vi "LIA Example Host_v1.vi"() -> ()   [LabVIEW 2017]
uses:
  Program Files (x86)/National Instruments/LabVIEW 2017/examples/Lock-In Amplifier/lib/host/Public/pll settings.ctl
  Program Files (x86)/National Instruments/LabVIEW 2017/examples/Lock-In Amplifier/lib/host/Public/lock-in settings.ctl
  Program Files (x86)/National Instruments/LabVIEW 2017/examples/Lock-In Amplifier/lib/interface/Interface FPGA/LIA Host Interface FPGA.lvclass
  C:/Program Files (x86)/National Instruments/LabVIEW 2017/examples/Lock-In Amplifier/lib/interface/Interface/LIA Host Interface.lvclass
  Program Files (x86)/National Instruments/LabVIEW 2017/examples/Lock-In Amplifier/lib/host/Public/fpga type.ctl
  Program Files (x86)/National Instruments/LabVIEW 2017/examples/Lock-In Amplifier/lib/interface/Interface FPGA/Properties/FpgaSession_GET.vi
  <vilib>/Utility/error.llb/Error Cluster From Error Code.vi
  <vilib>/rvi/errors/niLvFpgaAdjustHostInterfaceError.vi
  <vilib>/rvi/interface/nirviReadWriteControl/nirviReadWriteControl.xnode
  Program Files (x86)/National Instruments/LabVIEW 2017/examples/Lock-In Amplifier/lib/interface/Interface/LIA Host Interface.lvclass
  Program Files (x86)/National Instruments/LabVIEW 2017/examples/Lock-In Amplifier/lib/host/Lock-In Amplifier Example Host.lvlib
  Program Files (x86)/National Instruments/LabVIEW 2017/examples/Lock-In Amplifier/lib/shared/Lock-In Amplifier Example Shared.lvlib
  NiFpgaLv.dll
  <vilib>/rvi/interface/Simulation/niFpgaSimulationCallBeginRW.vi
panel:
  out "lock-in.max-min":dbl=7.228629495115158e-05 caption="Deviation" format="%#_6p"
  out "lock-in.max 0":dbl=0.9100438567932344 caption="Deviation" format="%#_6p"
  out "lock-in.min 0":dbl=0.9099715704982833 caption="Deviation" format="%#_6p"
  out "# of IQ samples":i32=4096 caption="Result"
  out "Waveform Chart":cluster{"mean":dbl, "trace":dbl}(graph)={"mean"=0.9100080307156506, "trace"=0.9100209129308812}
  out "Waveform Graph":cluster{"f0":dbl, "df":dbl, "magnitude":dbl[]}[](graph)
  in  "trigger slope 1":enum16{"Positive", "Negative"}(ring)
  in  "lowLevel 1":dbl caption="pll.q 2" format="%#_6f"
  in  "highLevel 1":dbl=0.25 caption="pll.q 2" format="%#_6f"
  in  "trigger slope 0":enum16{"Positive", "Negative"}(ring)
  in  "lowLevel 0":dbl caption="pll.q 2" format="%#_6f"
  in  "highLevel 0":dbl=0.25 caption="pll.q 2" format="%#_6f"
  out "pll.vco output 0":fxp<+/-,49,1>=0.001000059403974518 format="%0^#1_8g"
  out "pll.q 2":dbl=100005.9403974518 format="%#_6pV"
  in  "app.quit":bool
  in  "lock-in.boxcar length 0":u32=2048 caption="Boxar Length"
  in  "app.tab 0":enum32{"Lock-In", "PLL", "Output"}(tab)
  in  "lock-in.manual carrier 0":dbl=100000.0 caption="Carrier" format="%#_6p"
  in  "lock-in.decimation 0":i32=1000 caption="Decimation" min=8 max=16384
  in  "lock-in.source 0":enum16{"AI 0", "AI 1", "AI 2", "AI 3"}(ring)=enum."AI 1" caption="Channel"
  in  "lock-in.carrier 0":T1(ring)=enum."PLL 0" caption="Carrier Source"
  in  "pll.m 0":i8=-27 caption="M"
  in  "pll.source 0":enum16{"AI 0", "AI 1", "AI 2", "AI 3"}(ring) caption="Source"
  in  "pll.q frequency 0":dbl=100000.0 caption="Q Frequency" format="%#_6p"
  in  "pll.reset 0":bool
  in  "ao.noise 3":dbl caption="A0 3 Noise" min=0.0 max=1.0 format="%#_6p"
  in  "ao.level 3":dbl caption="A0 3 Level" format="%#_6pV"
  in  "ao.frequency 3":dbl=10000000.0 caption="AO 3 Frequency" format="%#.9p"
  in  "ao.frequency 0":dbl=10000000.0 caption="AO 0 Frequency" format="%#.9p"
  in  "ao.level 0":dbl caption="AO 0 Level" format="%#_6pV"
  in  "rio device":tag="PXI1Slot8" caption="Resource"
  in  "lock-in.reset boxar 0":bool
  out "lock-in.deviation 0":dbl=2.8087799509727284e-06 caption="Deviation" format="%#_6p"
  out "lock-in.amplitude 0":dbl=0.9100080307156506 caption="Result" format="%#_6p"
  in  "lock-in.boxcar lookback 0":i32=1024 caption="Windows to Average"
  # "pll.digital config 0"
  # "pll.digital config 1"
  # "NI Lock-In Amplifier Reference Example"
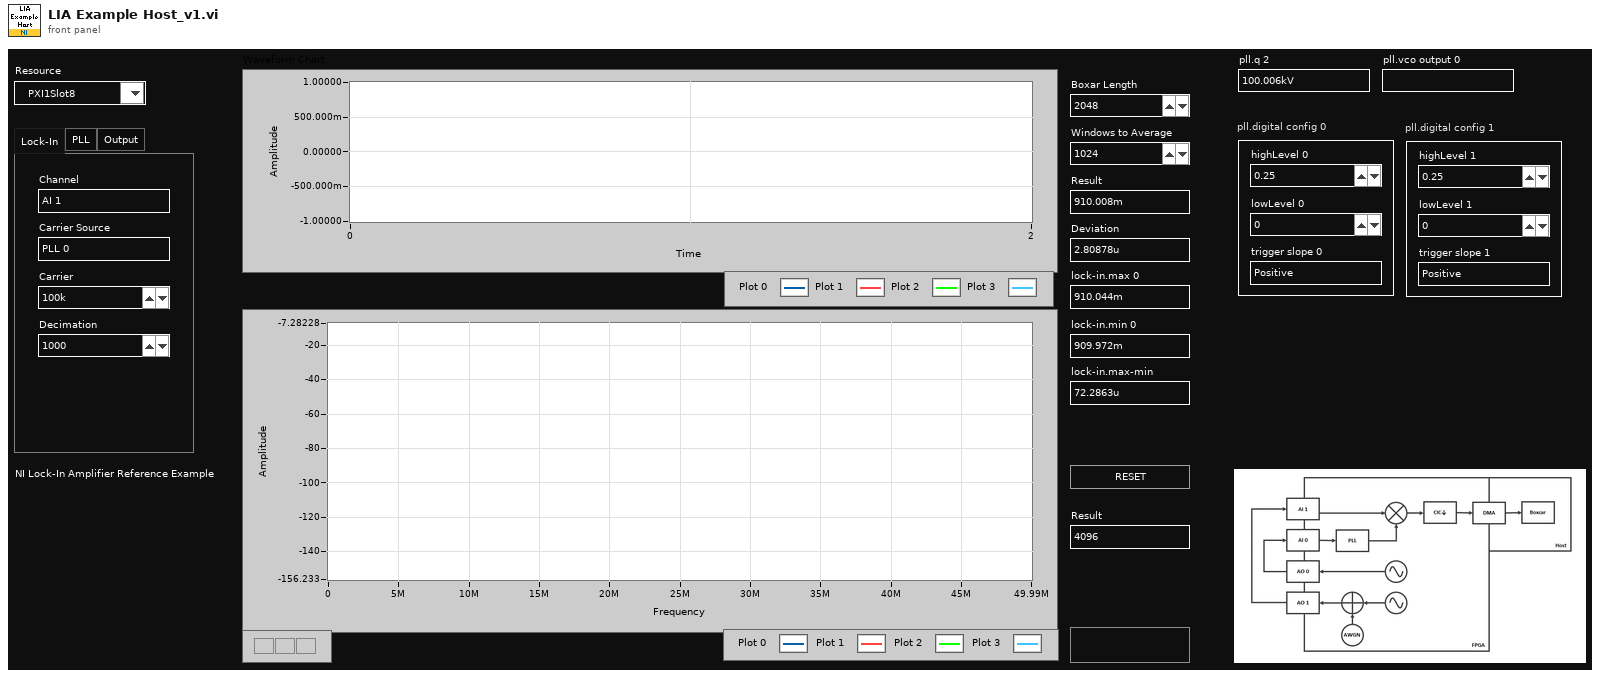
[diagram p1: front panel]
types:
  T1 = enum16{"Manual 0", "Manual 1", "Manual 2", "Manual 3", "PLL 0", "PLL 1"}
  T2 = typedef "Lock-In Amplifier Example Host.lvlib/lock-in settings.ctl" = cluster{"decimation":i32, "source":i32, "carrier source":i32, "carrier":dbl}
  T3 = typedef "Lock-In Amplifier Example Host.lvlib/pll settings.ctl" = cluster{"source":i32, "q frequency":dbl}
  T4 = cluster{"highLevel":fxp<+/-,18,1>, "lowLevel":fxp<+/-,18,1>, "trigger slope":enum8{"Positive", "Negative"}}
  T5 = typedef "Lock-In Amplifier Example Host.lvlib/fpga type.ctl" = refnum<k20>
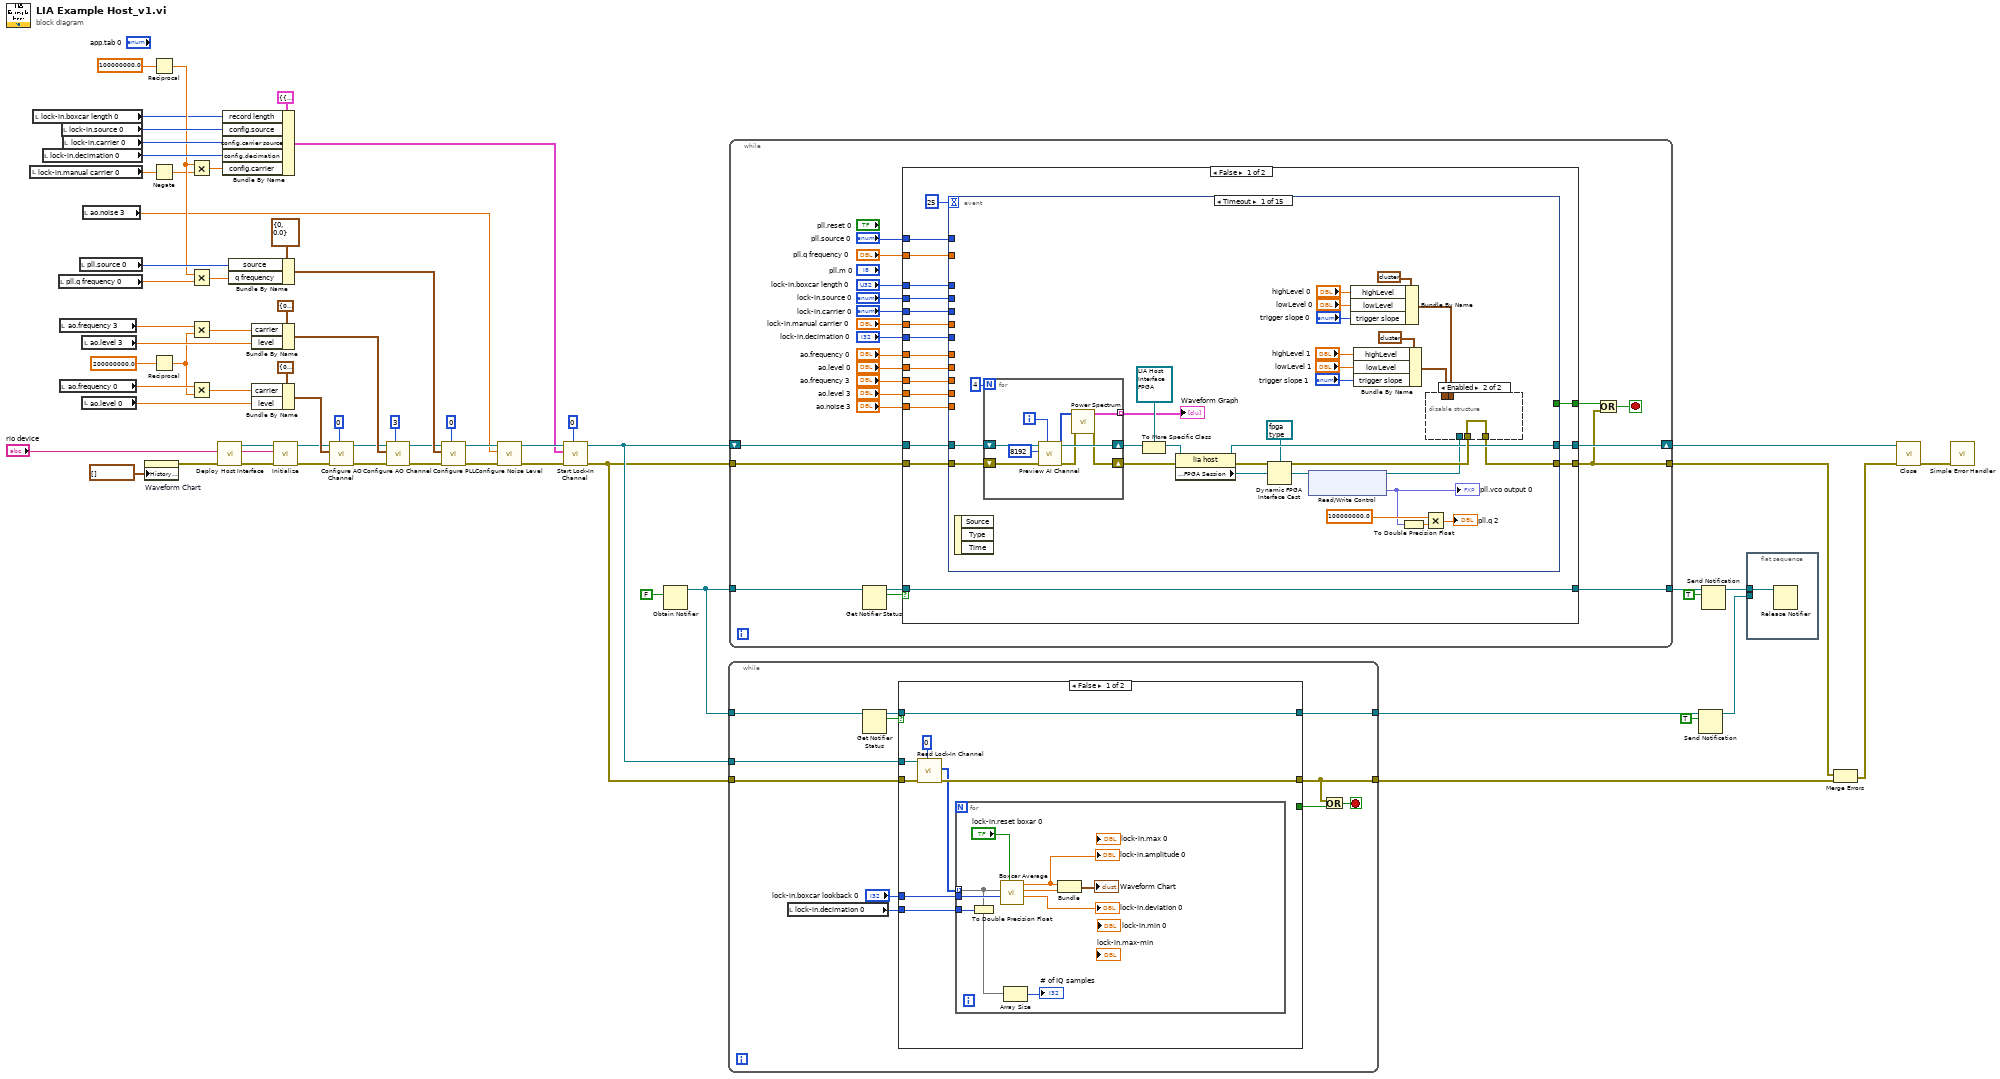
[diagram p0: block diagram]
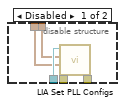
[diagram p2: hidden frame]
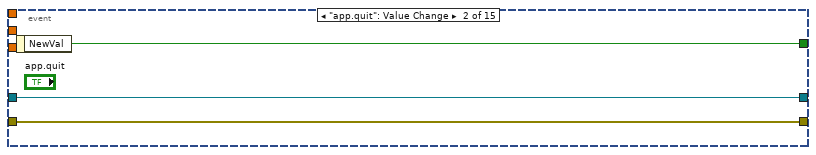
[diagram p3: hidden frame]
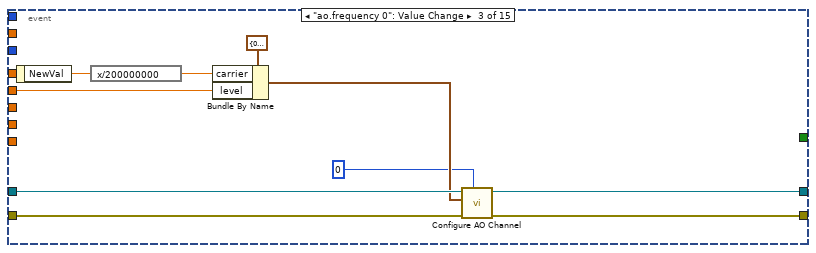
[diagram p4: hidden frame]
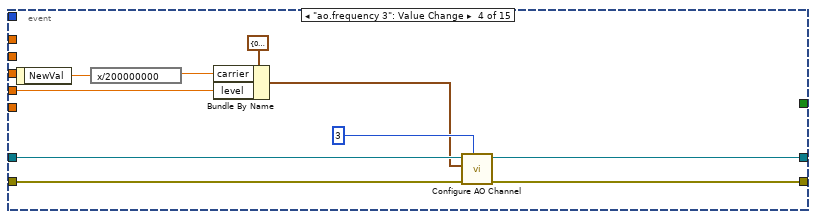
[diagram p5: hidden frame]
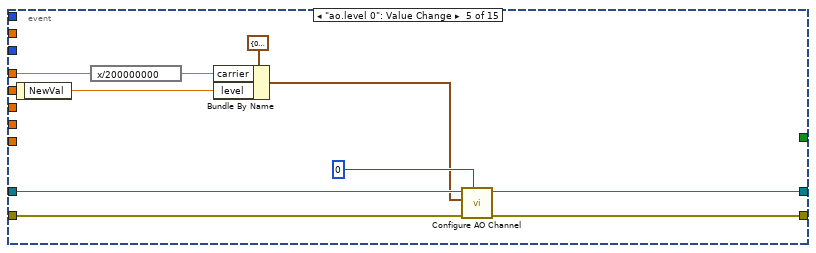
[diagram p6: hidden frame]
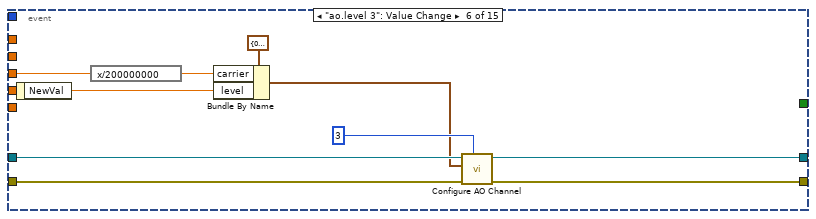
[diagram p7: hidden frame]
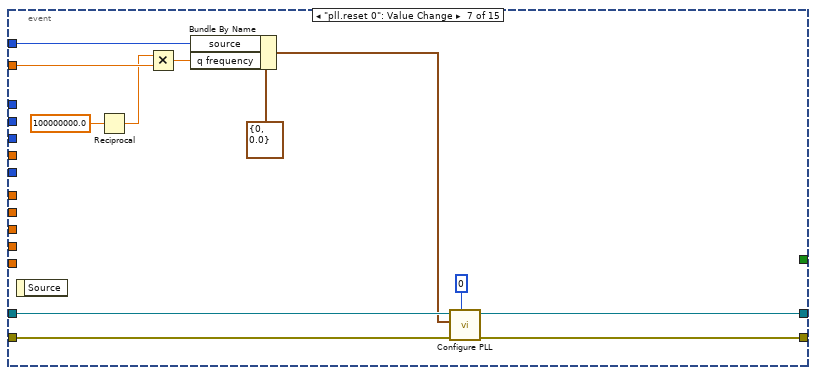
[diagram p8: hidden frame]
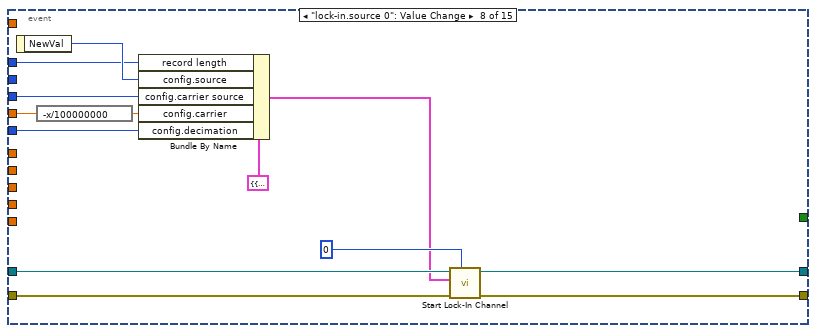
[diagram p9: hidden frame]
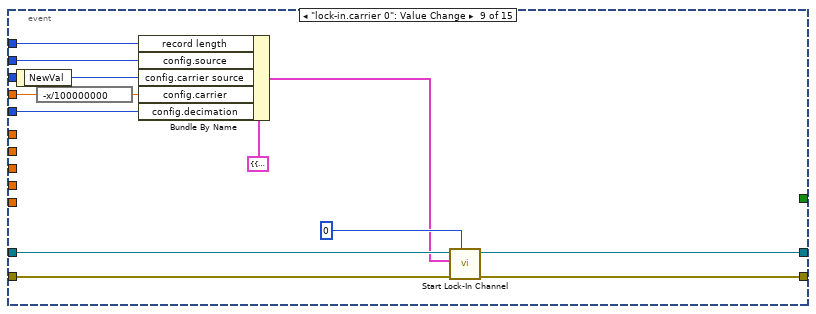
[diagram p10: hidden frame]
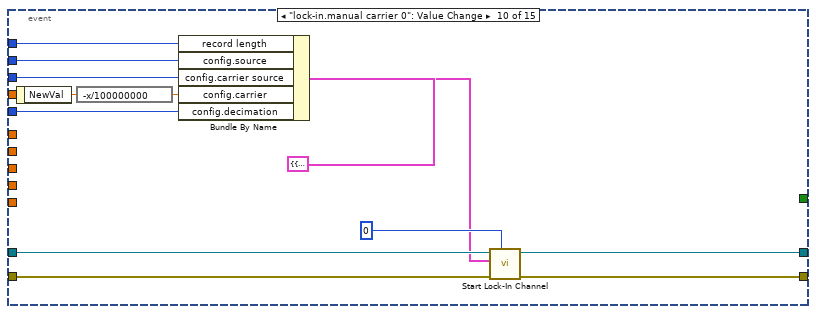
[diagram p11: hidden frame]
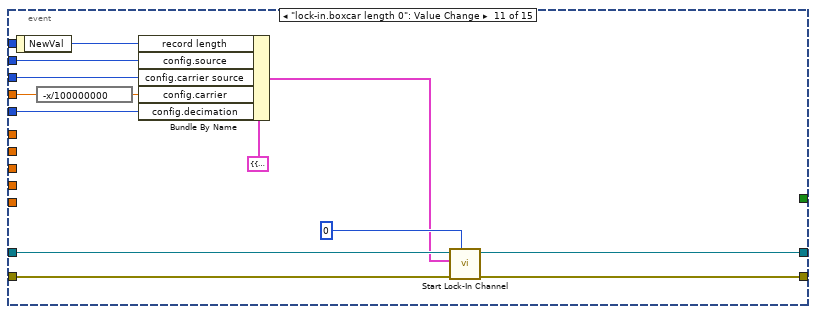
[diagram p12: hidden frame]
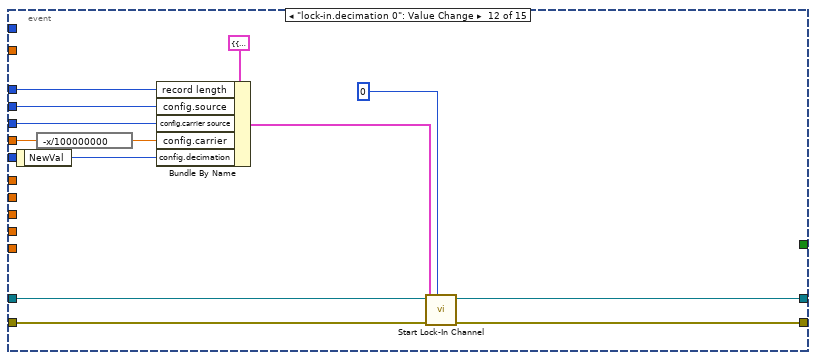
[diagram p13: hidden frame]
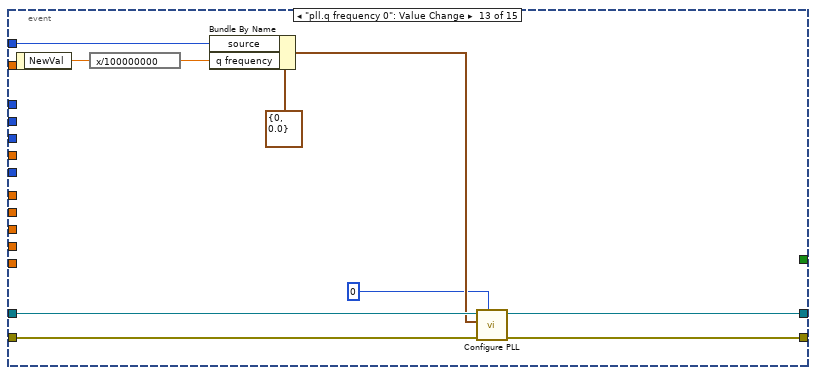
[diagram p14: hidden frame]
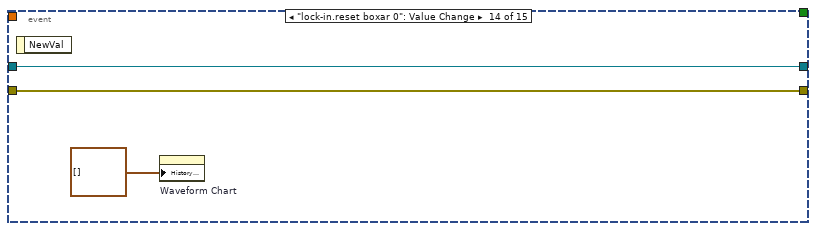
[diagram p15: hidden frame]
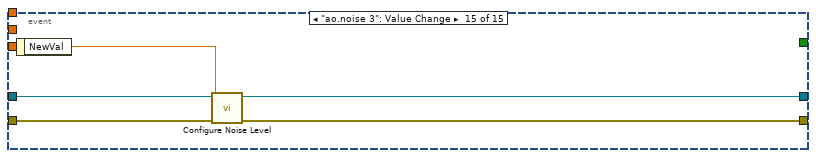
[diagram p16: hidden frame]
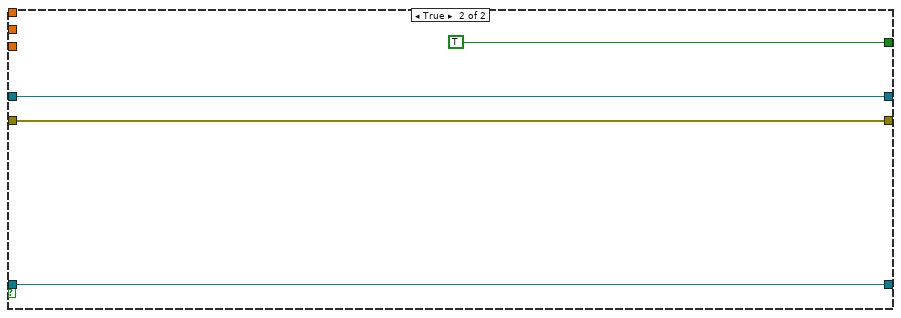
[diagram p17: hidden frame]
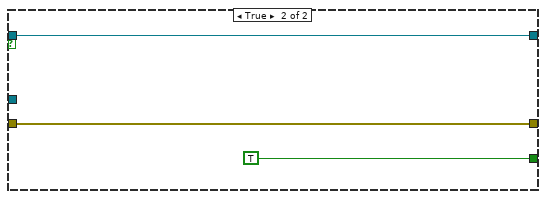
[diagram p18: hidden frame]
diagram:
  n1 = local read "lock-in.manual carrier 0"() -> (w50:dbl)
  n2 = local read "lock-in.boxcar length 0"() -> (w15:u32)
  n3 = local read "lock-in.decimation 0"() -> (w53:i32)
  n4 = local read "pll.q frequency 0"() -> (w55:dbl)
  n5 = local read "ao.frequency 3"() -> (w47:dbl)
  n6 = local read "ao.frequency 0"() -> (w44:dbl)
  n7 = local read "lock-in.source 0"() -> (w64:enum16{"AI 0", "AI 1", "AI 2", "AI 3"})
  n8 = local read "lock-in.carrier 0"() -> (w63:T1)
  n9 = local read "pll.source 0"() -> (w61:enum16{"AI 0", "AI 1", "AI 2", "AI 3"})
  n10 = local read "ao.level 3"() -> (w59:dbl)
  n11 = local read "ao.level 0"() -> (w58:dbl)
  n12 = local read "ao.noise 3"() -> (w6:dbl)
  n13 = property on="Waveform Chart" class="WFChart (strict)"("History Data"=cluster{"mean":dbl, "trace":dbl}[] []) -> (error out=w2:errorcluster)  [unwired: 2 in, 1 out]
  n14 = Reciprocal(x=100000000.0) -> (1/x=w51:dbl)
  n15 = Negate(x=w50) -> (-x=w49:dbl)
  n16 = Reciprocal(x=200000000.0) -> (1/x=w43:dbl)
  n17 = Multiply(x=w51, y=w49) -> (x*y=w52:dbl)
  n18 = Multiply(x=w51, y=w55) -> (x*y=w56:dbl)
  n19 = Multiply(x=w47, y=w43) -> (x*y=w48:dbl)
  n20 = Multiply(x=w44, y=w43) -> (x*y=w45:dbl)
  n21 = call "Deploy Host Interface.vi"("error in"=w2, "resource"="rio device") -> ("error out"=w11:errorcluster, "resource out"=w12:string, "lia host interface"=w13:refnum<class "LIA Host Interface.lvclass">)  [unwired: 7 in]
  n22 = Bundle By Name(cluster=cluster{"config":T2, "record length":u32} {"config"={"decimation"=0, "source"=0, "carrier source"=0, "carrier"=0.0}, "record length"=0} ("config"), "record length"=w15, "config.source"=w64, "config.carrier source"=w63, "config.decimation"=w53, "config.carrier"=w52) -> (w1:cluster{"config":T2, "record length":u32})
  n23 = Bundle By Name(cluster=T3 {"source"=0, "q frequency"=0.0} ("config"), "source"=w61, "q frequency"=w56) -> (w40:T3)
  n24 = Bundle By Name(cluster=cluster{"carrier":dbl, "level":dbl} {"carrier"=0.0, "level"=0.0} ("config"), "carrier"=w48, "level"=w59) -> (w41:cluster{"carrier":dbl, "level":dbl})
  n25 = Bundle By Name(cluster=cluster{"carrier":dbl, "level":dbl} {"carrier"=0.0, "level"=0.0} ("config"), "carrier"=w45, "level"=w58) -> (w42:cluster{"carrier":dbl, "level":dbl})
  n26 = call-dynamic "Initialize.vi"("error in"=w11, "resource"=w12, "lia host in"=w13) -> ("error out"=w24:errorcluster, "lia host out"=w25:refnum<class "LIA Host Interface.lvclass">)  [unwired: 7 in]
  n27 = call-dynamic "Configure AO Channel.vi"("instance"=0 ("index"), "error in"=w24, "config"=w42, "lia host in"=w25) -> ("error out"=w23:errorcluster, "lia host out"=w22:refnum<class "LIA Host Interface.lvclass">)  [unwired: 6 in]
  n28 = call-dynamic "Configure AO Channel.vi"("instance"=3 ("index"), "error in"=w23, "config"=w41, "lia host in"=w22) -> ("error out"=w18:errorcluster, "lia host out"=w19:refnum<class "LIA Host Interface.lvclass">)  [unwired: 6 in]
  n29 = call-dynamic "Configure PLL.vi"("instance"=0 ("index"), "error in"=w18, "config"=w40, "lia host in"=w19) -> ("error out"=w10:errorcluster, "lia host out"=w7:refnum<class "LIA Host Interface.lvclass">)  [unwired: 6 in]
  n30 = call-dynamic "Configure Noise Level.vi"("error in"=w10, "level"=w6, "lia host in"=w7) -> ("error out"=w9:errorcluster, "lia host out"=w8:refnum<class "LIA Host Interface.lvclass">)  [unwired: 7 in]
  n31 = call-dynamic "Start Lock-In Channel.vi"("instance"=0 ("index"), "error in"=w9, "config"=w1, "lia host in"=w8) -> ("error out"=w35:errorcluster, "lia host out"=w36:refnum<class "LIA Host Interface.lvclass">)  [unwired: 6 in]
  n32 = Obtain Notifier(notification data type=FALSE) -> (notifier out=w37:refnum<notifier>)  [unwired: 3 in, 2 out]
  n33 = while {
    tunnel: w37 -> [w75]
    tunnel: w36 -> [w72]
    tunnel: w35 -> [w71]
    tunnel: [w70] -> w28
    tunnel: [w67] -> w31
    stop <- w69 stop-if-true
    n34 = local read "lock-in.decimation 0"() -> (w65:i32)
    n35 = Get Notifier Status(notifier=w75) -> (notifier out=w73:refnum<notifier>, current notification=w74:bool)  [unwired: 1 in, 3 out]
    n36 = case shown="False" w74 {
      tunnel: [w80 w95] -> w67
      tunnel: w73 -> [w80 w95]
      tunnel: w72 -> [w83 _]
      tunnel: w71 -> [w82 w94]
      tunnel: [w79 w94] -> w70
      tunnel: [_ TRUE] -> w68
      tunnel: "lock-in.boxcar lookback 0" -> [w78 _]
      tunnel: w65 -> [w76 _]
      frame False {
        n37 = call-dynamic "Read Lock-In Channel.vi"("instance"=0 ("index"), "error in"=w82, "lia host in"=w83) -> ("error out"=w79:errorcluster, "unscaled data"=w77:i64[][])  [unwired: 6 in, 1 out]
        n38 = for {
          tunnel: w77 -> [w85] mode=indexing
          tunnel: w78 -> [w90]
          tunnel: w76 -> [w84]
          n39 = To Double Precision Float(number=w84) -> ()  [unwired: 1 out]
          n40 = call "Boxcar Average.vi"("reset"="lock-in.reset boxar 0", "sample length"=w90, "interleaved iq"=w85) -> ("standard deviation"=→"lock-in.deviation 0":dbl, "trace"=w87:dbl, "mean"=w91:dbl)  [unwired: 6 in]
          "lock-in.amplitude 0" <- w91
          n41 = Array Size(array=w85) -> (size(s)=→"# of IQ samples":i32)
          n42 = Bundle("mean"=w91, "trace"=w87) -> (→"Waveform Chart":cluster{"mean":dbl, "trace":dbl})  [unwired: 1 in]
        }
      }
      frame True {
      }
    }
    n43 = Or(x=w70, y=w68) -> (x .or. y?=w69:bool)
  }
  n44 = while {
    tunnel: w35 -> [w117]
    shift-right: [w103] -> w39
    shift-left: w36 -> [w116]
    tunnel: [w99] -> w27
    tunnel: w37 -> [w102]
    tunnel: [w97] -> w34
    stop <- w115 stop-if-true
    n45 = Get Notifier Status(notifier=w102) -> (notifier out=w101:refnum<notifier>, current notification=w100:bool)  [unwired: 1 in, 3 out]
    n46 = case shown="False" w100 {
      tunnel: w117 -> [w136 w321]
      tunnel: w116 -> [w135 w322]
      tunnel: [w134 w321] -> w99
      tunnel: "lock-in.manual carrier 0" -> [w132 _]
      tunnel: "lock-in.decimation 0" -> [w131 _]
      tunnel: "lock-in.source 0" -> [w130 _]
      tunnel: "lock-in.carrier 0" -> [w129 _]
      tunnel: "pll.source 0" -> [w128 _]
      tunnel: "pll.q frequency 0" -> [w127 _]
      tunnel: "ao.frequency 0" -> [w126 _]
      tunnel: "ao.level 0" -> [w125 _]
      tunnel: "ao.frequency 3" -> [w124 _]
      tunnel: "ao.level 3" -> [w123 _]
      tunnel: "ao.noise 3" -> [w122 _]
      tunnel: [w121 w322] -> w103
      tunnel: w101 -> [w119 w319]
      tunnel: [w120 TRUE] -> w98
      tunnel: [w119 w319] -> w97
      tunnel: "lock-in.boxcar length 0" -> [w118 _]
      frame False {
        n47 = event shown="[0] Timeout" {
          selector: _ -> [_ _ _ _ _ _ _ _ _ _ _ _ _ _ _]
          dyn-events: _ -> [_ _ _ _ _ _ _ _ _ _ _ _ _ _ _]
          timeout: 25 -> [_ _ _ _ _ _ _ _ _ _ _ _ _ _ _]
          tunnel: w136 -> [w163 w182 w188 w203 w213 w223 w235 w244 w258 w271 w283 w297 w306 w312 w317]
          tunnel: w135 -> [w164 w183 w189 w202 w212 w222 w234 w242 w256 w269 w281 w295 w305 w313 w318]
          tunnel: [w154 w182 w186 w201 w211 w221 w233 w243 w257 w270 w282 w296 w303 w312 w315] -> w134
          tunnel: w130 -> [_ _ _ _ _ _ _ _ w249 w262 w275 w291 _ _ _]
          tunnel: w129 -> [_ _ _ _ _ _ _ w247 _ w273 w286 w299 _ _ _]
          tunnel: w132 -> [_ _ _ _ _ _ _ w246 w260 _ w285 w298 _ _ _]
          tunnel: w131 -> [_ _ _ _ _ _ _ w245 w259 w272 w284 _ _ _ _]
          tunnel: w128 -> [_ _ _ _ _ _ w228 _ _ _ _ _ w308 _ _]
          tunnel: w127 -> [_ _ _ _ _ _ w229 _ _ _ _ _ _ _ _]
          tunnel: w126 -> [_ _ _ _ w206 _ _ _ _ _ _ _ _ _ _]
          tunnel: w125 -> [_ _ w191 _ _ _ _ _ _ _ _ _ _ _ _]
          tunnel: w124 -> [_ _ _ _ _ w216 _ _ _ _ _ _ _ _ _]
          tunnel: w123 -> [_ _ _ w196 _ _ _ _ _ _ _ _ _ _ _]
          tunnel: w122 -> [_ _ _ _ _ _ _ _ _ _ _ _ _ _ _]
          tunnel: [w159 w183 w184 w194 w204 w214 w224 w241 w255 w268 w280 w294 w304 w313 w316] -> w121
          tunnel: [_ w181 _ _ _ _ _ _ _ _ _ _ _ _ _] -> w120
          tunnel: w118 -> [_ _ _ _ _ _ _ w237 w252 w265 _ w289 _ _ _]
          event Timeout {
            n48 = event-data() -> ()  [unwired: 1 in, 3 out]
            n49 = for {
              N: 4 -> [_]
              shift-right: [w178] -> w160
              shift-left: w164 -> [w180]
              shift-right: [w176] -> w162
              shift-left: w163 -> [w179]
              tunnel: [w174] -> w137 mode=indexing
              i -> [w172]
              n50 = call-dynamic "Preview AI Channel.vi"("instance"=w172, "error in"=w179, "samples"=u32 8192, "lia host in"=w180) -> ("error out"=w177:errorcluster, "samples"=w175:i16[], "lia host out"=w178:refnum<class "LIA Host Interface.lvclass">)  [unwired: 5 in]
              n51 = call "Power Spectrum.vi"("error in"=w177, "ai data"=w175) -> ("error out"=w176:errorcluster, "magnitude"=w174:cluster{"f0":dbl, "df":dbl, "magnitude":dbl[]})  [unwired: 8 in]
            }
            "Waveform Graph" <- w137
            n52 = To More Specific Class(target class=refnum<class "LIA Host Interface FPGA.lvclass"> refnum ("lia host"), reference=w160) -> (specific class reference=w158:refnum<class "LIA Host Interface FPGA.lvclass">)  [unwired: 1 in, 1 out]
            n53 = property class="lia host"(reference=w158, error in=w162) -> (reference out=w159:refnum<class "LIA Host Interface FPGA.lvclass">, error out=w165:errorcluster, "Properties:FPGA Session"=w156:refnum<k20>)
            n54 = Dynamic FPGA Interface Cast(Session In=T5 refnum ("fpga type"), Type=w156) -> (Session Out=w153:T5)
            n55 = xnode "Read/Write Control"("FPGA VI Reference In"=w153) -> ("FPGA VI Reference Out"=w149:T5, "pll.vco output 0"=w148:fxp<+/-,48,0>)  [unwired: 1 in, 1 out]
            "pll.vco output 0" <- w148
            n56 = Bundle By Name(cluster=T4 {"highLevel"=0.0, "lowLevel"=0.0, "trigger slope"=enum."Positive"} ("pll.digital config 0"), "highLevel"="highLevel 0", "lowLevel"="lowLevel 0", "trigger slope"="trigger slope 0") -> (w139:T4)
            n57 = Bundle By Name(cluster=T4 {"highLevel"=0.0, "lowLevel"=0.0, "trigger slope"=enum."Positive"} ("pll.digital config 0"), "highLevel"="highLevel 1", "lowLevel"="lowLevel 1", "trigger slope"="trigger slope 1") -> (w138:T4)
            n58 = To Double Precision Float(number=w148) -> (double precision float=w152:dbl)
            n59 = Multiply(x=100000000.0, y=w152) -> (x*y=→"pll.q 2":dbl)
            n60 = disable-structure shown="Enabled" {
              disable-tunnel: w165 -> [w170 w171]
              disable-tunnel: [w169 w171] -> w154
              disable-tunnel: w149 -> [w168 _]
              disable-tunnel: w139 -> [w167 _]
              disable-tunnel: w138 -> [w166 _]
              frame Disabled {
                n61 = call "LIA Set PLL Configs.vi"("error in (no error)"=w170, "pll.digital config 1"=w166, "pll.digital config 0"=w167, "fpga session in"=w168) -> ("error out"=w169:errorcluster)  [unwired: 7 in]
              }
              frame Enabled {
              }
            }
          }
          event "app.quit": Value Change {
            n62 = event-data() -> ("NewVal"=w181:bool)  [unwired: 1 in]
          }
          event "ao.frequency 0": Value Change {
            n63 = event-data() -> ("NewVal"=w190:dbl)  [unwired: 1 in]
            n64 = expression code="x/200000000"(w190) -> (w192:dbl)
            n65 = Bundle By Name(cluster=cluster{"carrier":dbl, "level":dbl} {"carrier"=0.0, "level"=0.0} ("config"), "carrier"=w192, "level"=w191) -> (w187:cluster{"carrier":dbl, "level":dbl})
            n66 = call-dynamic "Configure AO Channel.vi"("instance"=0 ("index"), "error in"=w188, "config"=w187, "lia host in"=w189) -> ("error out"=w186:errorcluster, "lia host out"=w184:refnum<class "LIA Host Interface.lvclass">)  [unwired: 6 in]
          }
          event "ao.frequency 3": Value Change {
            n67 = event-data() -> ("NewVal"=w197:dbl)  [unwired: 1 in]
            n68 = expression code="x/200000000"(w197) -> (w199:dbl)
            n69 = Bundle By Name(cluster=cluster{"carrier":dbl, "level":dbl} {"carrier"=0.0, "level"=0.0} ("config"), "carrier"=w199, "level"=w196) -> (w195:cluster{"carrier":dbl, "level":dbl})
            n70 = call-dynamic "Configure AO Channel.vi"("instance"=3 ("index"), "error in"=w203, "config"=w195, "lia host in"=w202) -> ("error out"=w201:errorcluster, "lia host out"=w194:refnum<class "LIA Host Interface.lvclass">)  [unwired: 6 in]
          }
          event "ao.level 0": Value Change {
            n71 = event-data() -> ("NewVal"=w207:dbl)  [unwired: 1 in]
            n72 = expression code="x/200000000"(w206) -> (w209:dbl)
            n73 = Bundle By Name(cluster=cluster{"carrier":dbl, "level":dbl} {"carrier"=0.0, "level"=0.0} ("config"), "carrier"=w209, "level"=w207) -> (w205:cluster{"carrier":dbl, "level":dbl})
            n74 = call-dynamic "Configure AO Channel.vi"("instance"=0 ("index"), "error in"=w213, "config"=w205, "lia host in"=w212) -> ("error out"=w211:errorcluster, "lia host out"=w204:refnum<class "LIA Host Interface.lvclass">)  [unwired: 6 in]
          }
          event "ao.level 3": Value Change {
            n75 = event-data() -> ("NewVal"=w217:dbl)  [unwired: 1 in]
            n76 = expression code="x/200000000"(w216) -> (w219:dbl)
            n77 = Bundle By Name(cluster=cluster{"carrier":dbl, "level":dbl} {"carrier"=0.0, "level"=0.0} ("config"), "carrier"=w219, "level"=w217) -> (w215:cluster{"carrier":dbl, "level":dbl})
            n78 = call-dynamic "Configure AO Channel.vi"("instance"=3 ("index"), "error in"=w223, "config"=w215, "lia host in"=w222) -> ("error out"=w221:errorcluster, "lia host out"=w214:refnum<class "LIA Host Interface.lvclass">)  [unwired: 6 in]
          }
          event "pll.reset 0": Value Change {
            n79 = event-data() -> ()  [unwired: 1 in, 1 out]
            n80 = Reciprocal(x=100000000.0) -> (1/x=w226:dbl)
            n81 = Multiply(x=w226, y=w229) -> (x*y=w231:dbl)
            n82 = Bundle By Name(cluster=T3 {"source"=0, "q frequency"=0.0} ("config"), "source"=w228, "q frequency"=w231) -> (w225:T3)
            n83 = call-dynamic "Configure PLL.vi"("instance"=0 ("index"), "error in"=w235, "config"=w225, "lia host in"=w234) -> ("error out"=w233:errorcluster, "lia host out"=w224:refnum<class "LIA Host Interface.lvclass">)  [unwired: 6 in]
          }
          event "lock-in.source 0": Value Change {
            n84 = event-data() -> ("NewVal"=w239:enum16{"AI 0", "AI 1", "AI 2", "AI 3"})  [unwired: 1 in]
            n85 = expression code="-x/100000000"(w246) -> (w248:dbl)
            n86 = Bundle By Name(cluster=cluster{"config":T2, "record length":u32} {"config"={"decimation"=0, "source"=0, "carrier source"=0, "carrier"=0.0}, "record length"=0} ("config"), "record length"=w237, "config.source"=w239, "config.carrier source"=w247, "config.carrier"=w248, "config.decimation"=w245) -> (w236:cluster{"config":T2, "record length":u32})
            n87 = call-dynamic "Start Lock-In Channel.vi"("instance"=0 ("index"), "error in"=w244, "config"=w236, "lia host in"=w242) -> ("error out"=w243:errorcluster, "lia host out"=w241:refnum<class "LIA Host Interface.lvclass">)  [unwired: 6 in]
          }
          event "lock-in.carrier 0": Value Change {
            n88 = event-data() -> ("NewVal"=w250:T1)  [unwired: 1 in]
            n89 = expression code="-x/100000000"(w260) -> (w261:dbl)
            n90 = Bundle By Name(cluster=cluster{"config":T2, "record length":u32} {"config"={"decimation"=0, "source"=0, "carrier source"=0, "carrier"=0.0}, "record length"=0} ("config"), "record length"=w252, "config.source"=w249, "config.carrier source"=w250, "config.carrier"=w261, "config.decimation"=w259) -> (w251:cluster{"config":T2, "record length":u32})
            n91 = call-dynamic "Start Lock-In Channel.vi"("instance"=0 ("index"), "error in"=w258, "config"=w251, "lia host in"=w256) -> ("error out"=w257:errorcluster, "lia host out"=w255:refnum<class "LIA Host Interface.lvclass">)  [unwired: 6 in]
          }
          event "lock-in.manual carrier 0": Value Change {
            n92 = event-data() -> ("NewVal"=w263:dbl)  [unwired: 1 in]
            n93 = expression code="-x/100000000"(w263) -> (w274:dbl)
            n94 = Bundle By Name(cluster=cluster{"config":T2, "record length":u32} {"config"={"decimation"=0, "source"=0, "carrier source"=0, "carrier"=0.0}, "record length"=0} ("config"), "record length"=w265, "config.source"=w262, "config.carrier source"=w273, "config.carrier"=w274, "config.decimation"=w272) -> (w264:cluster{"config":T2, "record length":u32})
            n95 = call-dynamic "Start Lock-In Channel.vi"("instance"=0 ("index"), "error in"=w271, "config"=w264, "lia host in"=w269) -> ("error out"=w270:errorcluster, "lia host out"=w268:refnum<class "LIA Host Interface.lvclass">)  [unwired: 6 in]
          }
          event "lock-in.boxcar length 0": Value Change {
            n96 = event-data() -> ("NewVal"=w276:u32)  [unwired: 1 in]
            n97 = expression code="-x/100000000"(w285) -> (w287:dbl)
            n98 = Bundle By Name(cluster=cluster{"config":T2, "record length":u32} {"config"={"decimation"=0, "source"=0, "carrier source"=0, "carrier"=0.0}, "record length"=0} ("config"), "record length"=w276, "config.source"=w275, "config.carrier source"=w286, "config.carrier"=w287, "config.decimation"=w284) -> (w277:cluster{"config":T2, "record length":u32})
            n99 = call-dynamic "Start Lock-In Channel.vi"("instance"=0 ("index"), "error in"=w283, "config"=w277, "lia host in"=w281) -> ("error out"=w282:errorcluster, "lia host out"=w280:refnum<class "LIA Host Interface.lvclass">)  [unwired: 6 in]
          }
          event "lock-in.decimation 0": Value Change {
            n100 = event-data() -> ("NewVal"=w292:i32)  [unwired: 1 in]
            n101 = expression code="-x/100000000"(w298) -> (w300:dbl)
            n102 = Bundle By Name(cluster=cluster{"config":T2, "record length":u32} {"config"={"decimation"=0, "source"=0, "carrier source"=0, "carrier"=0.0}, "record length"=0} ("config"), "record length"=w289, "config.source"=w291, "config.carrier source"=w299, "config.carrier"=w300, "config.decimation"=w292) -> (w288:cluster{"config":T2, "record length":u32})
            n103 = call-dynamic "Start Lock-In Channel.vi"("instance"=0 ("index"), "error in"=w297, "config"=w288, "lia host in"=w295) -> ("error out"=w296:errorcluster, "lia host out"=w294:refnum<class "LIA Host Interface.lvclass">)  [unwired: 6 in]
          }
          event "pll.q frequency 0": Value Change {
            n104 = event-data() -> ("NewVal"=w307:dbl)  [unwired: 1 in]
            n105 = expression code="x/100000000"(w307) -> (w310:dbl)
            n106 = Bundle By Name(cluster=T3 {"source"=0, "q frequency"=0.0} ("config"), "source"=w308, "q frequency"=w310) -> (w302:T3)
            n107 = call-dynamic "Configure PLL.vi"("instance"=0, "error in"=w306, "config"=w302, "lia host in"=w305) -> ("error out"=w303:errorcluster, "lia host out"=w304:refnum<class "LIA Host Interface.lvclass">)  [unwired: 6 in]
          }
          event "lock-in.reset boxar 0": Value Change {
            n108 = event-data() -> ()  [unwired: 1 in, 1 out]
            n109 = property on="Waveform Chart" class="WFChart (strict)"("History Data"=cluster{"mean":dbl, "trace":dbl}[] []) -> ()  [unwired: 2 in, 2 out]
          }
          event "ao.noise 3": Value Change {
            n110 = event-data() -> ("NewVal"=w314:dbl)  [unwired: 1 in]
            n111 = call-dynamic "Configure Noise Level.vi"("error in"=w317, "level"=w314, "lia host in"=w318) -> ("error out"=w315:errorcluster, "lia host out"=w316:refnum<class "LIA Host Interface.lvclass">)  [unwired: 7 in]
          }
        }
      }
      frame True {
      }
    }
    n112 = Or(x=w98, y=w99) -> (x .or. y?=w115:bool)
  }
  n113 = Send Notification(notification=TRUE, notifier=w31) -> (notifier out=w29:refnum<notifier>)  [unwired: 1 in, 1 out]
  n114 = Send Notification(notification=TRUE, notifier=w34) -> (notifier out=w30:refnum<notifier>)  [unwired: 1 in, 1 out]
  n115 = flat-sequence {
    tunnel: w30 -> [w323]
    tunnel: w29 -> [_]
    frame #0 {
      n116 = Release Notifier(notifier=w323) -> ()  [unwired: 2 in, 3 out]
    }
  }
  n117 = Merge Errors(w27, w28) -> (w26:errorcluster)
  n118 = call-dynamic "Close.vi"("error in"=w26, "lia host in"=w39) -> ("error out"=w5:errorcluster)  [unwired: 8 in, 1 out]
  n119 = call <vilib>:"Simple Error Handler.vi"("error in (no error)"=w5) -> ()  [unwired: 4 in, 5 out]
